vi "RemoveNode.vi"(8 "error in (no error)":errorcluster, 9 "position":T1, 11 "LinkedList in":refnum<class "LinkedList.lvclass">) -> (0 "error out":errorcluster, 1 "ignored":bool, 2 "RemovedNode":refnum<data-value>, 3 "LinkedList out":refnum<class "LinkedList.lvclass">)   [LabVIEW 2013, in "LinkedList.lvclass"]
doc: "Removes a single node from a linked list. If you choose the search option, you must override the IsGoalNode.vi to choose which node to remove."
uses:
  LinkedList.lvclass
  position.ctl
  LLNode/LLNode.lvclass
  LinkedList.lvclass/LinkedList.ctl
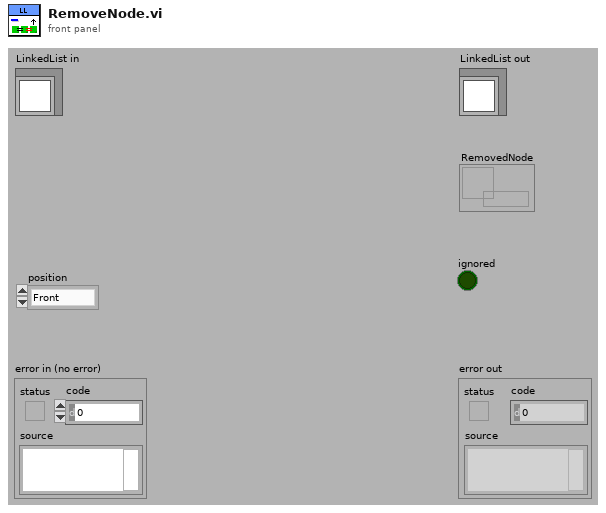
[diagram p1: front panel]
types:
  T1 = typedef "LinkedList.lvclass/position.ctl" = enum16{"Front", "Back", "Search"}
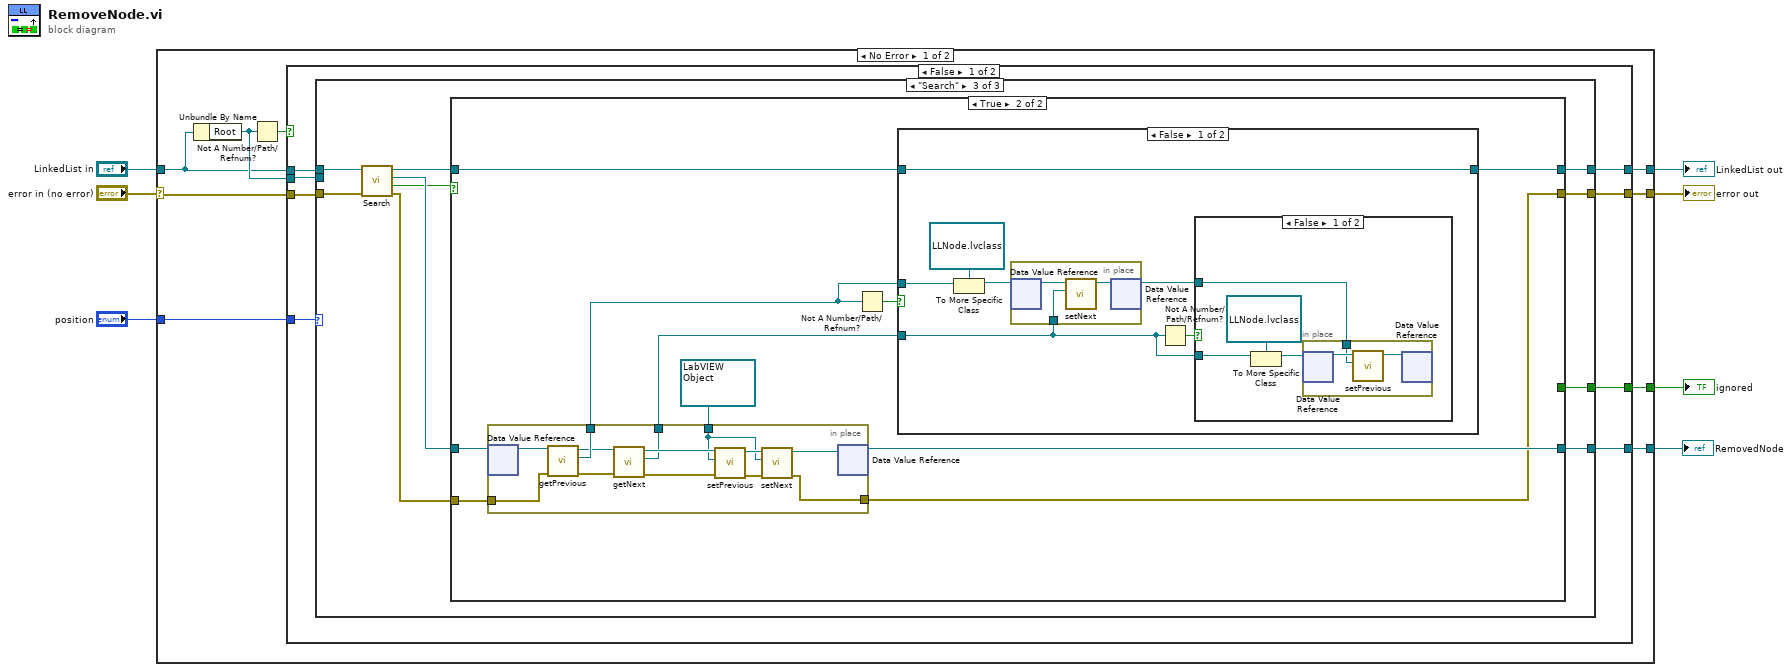
[diagram p0: block diagram]
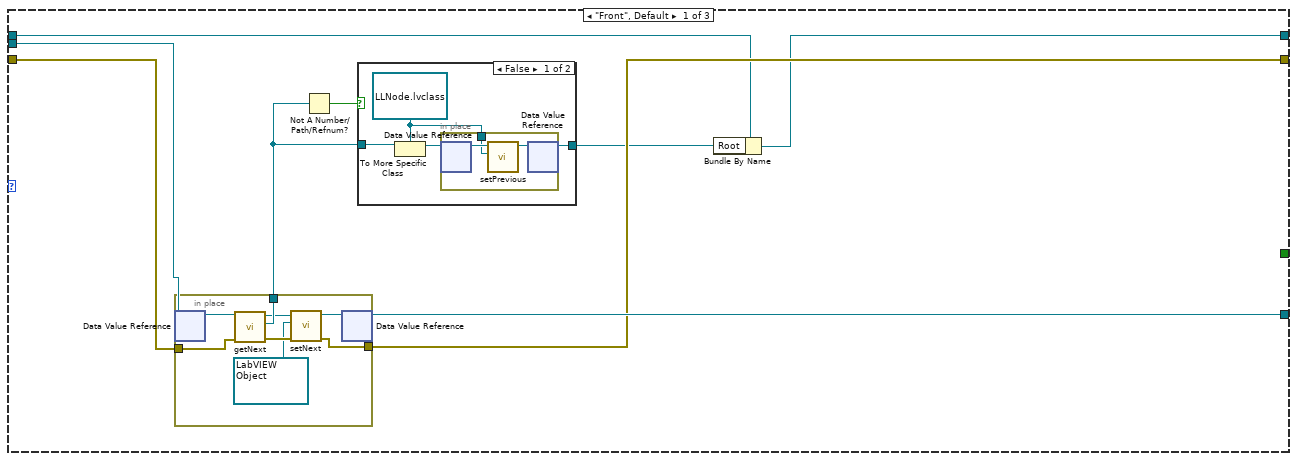
[diagram p2: hidden frame]
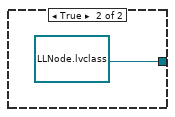
[diagram p3: hidden frame]
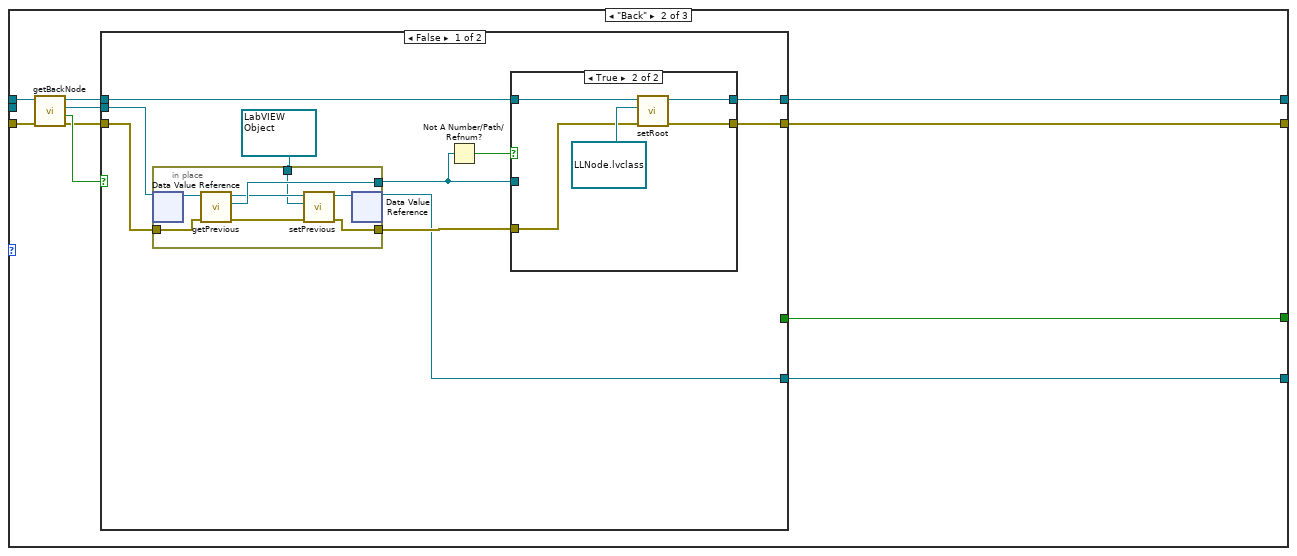
[diagram p4: hidden frame]
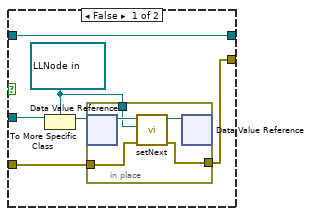
[diagram p5: hidden frame]
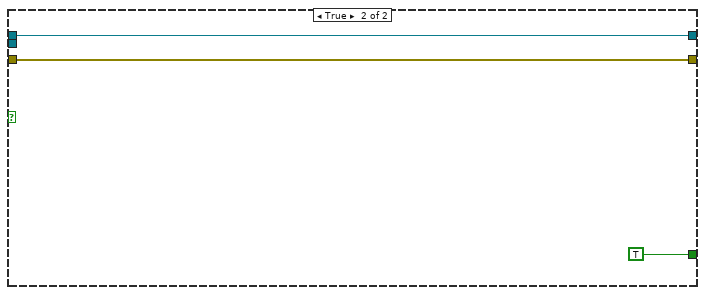
[diagram p6: hidden frame]
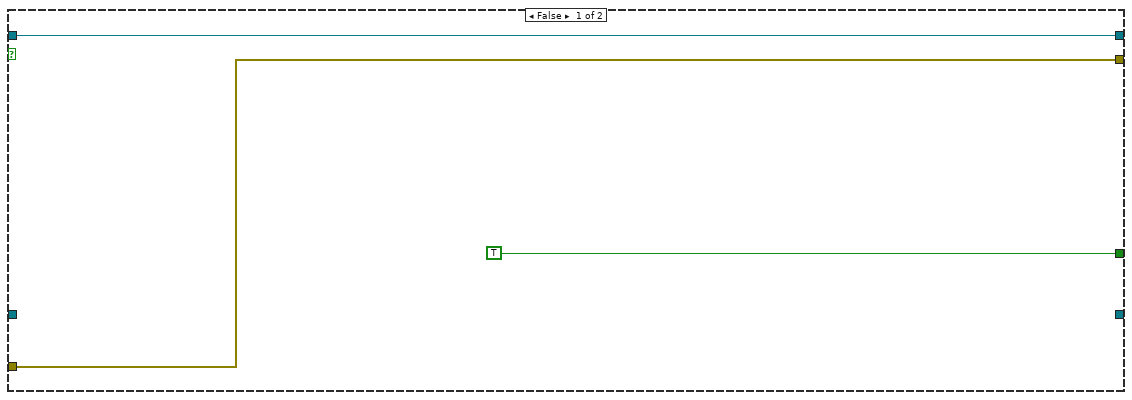
[diagram p7: hidden frame]
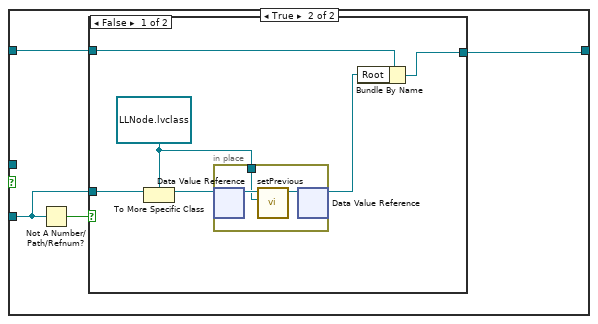
[diagram p9: hidden frame]
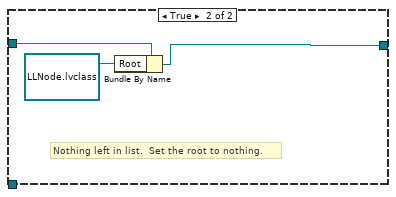
[diagram p10: hidden frame]
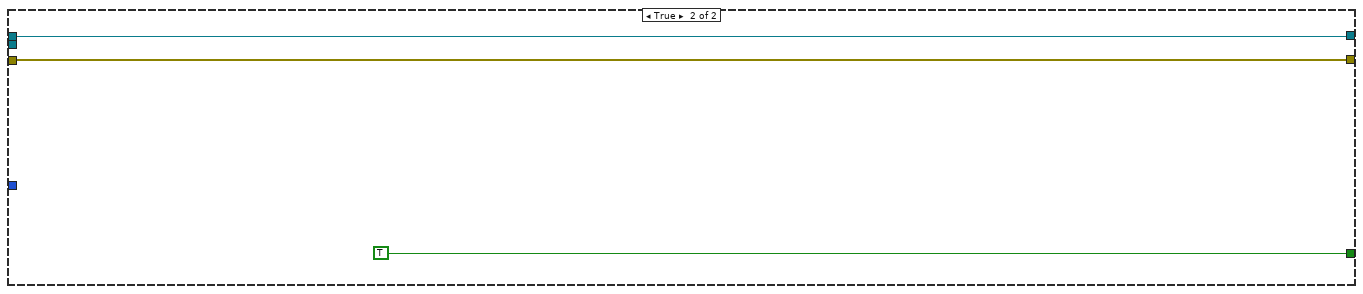
[diagram p11: hidden frame]
diagram:
  n1 = case shown="No Error" "error in (no error)" {
    selector: "error in (no error)" -> [w8 w170]
    tunnel: [w14 w170] -> w6
    tunnel: [w15 w169] -> w4
    tunnel: "LinkedList in" -> [w9 w169]
    tunnel: "position" -> [w16 _]
    tunnel: [w13 _] -> w2
    tunnel: [w12 _] -> w1
    frame No Error {
      n2 = Unbundle By Name(w9) -> ("Root"=w10:refnum<data-value>)
      n3 = Not A Number/Path/Refnum?(number/path/refnum=w10) -> (NaN/Path/Refnum?=w11:bool)
      n4 = case shown="False" w11 {
        tunnel: w16 -> [w24 _]
        tunnel: [w23 TRUE] -> w13
        tunnel: [w22 w168] -> w15
        tunnel: [w21 w167] -> w14
        tunnel: [w20 _] -> w12
        tunnel: w8 -> [w19 w167]
        tunnel: w9 -> [w18 w168]
        tunnel: w10 -> [w17 _]
        frame False {
          n5 = case shown="\"Search\"" w24 {
            tunnel: w18 -> [w27 w59 w102]
            tunnel: [_ w50 w106] -> w23
            tunnel: w19 -> [w32 w56 w100]
            tunnel: [w26 w53 w105] -> w22
            tunnel: [w28 w52 w104] -> w21
            tunnel: [w33 w51 w103] -> w20
            tunnel: w17 -> [w31 _ _]
            frame "Front", Default {
              n6 = in-place {
                in-place-border: w32 -> [w48]
                in-place-border: [w43] -> w28
                in-place-border: [w47] -> w29
                n7 = in-place-dvr #1(w31) -> (w49:refnum<class "LLNode.lvclass">)  [unwired: 1 out]
                n8 = call "getNext.vi"("error in (no error)"=w48, "LLNode in"=w49) -> ("error out"=w44:errorcluster, "next"=w47:refnum<data-value>, "LLNode out"=w46:refnum<class "LLNode.lvclass">)  [unwired: 7 in]
                n9 = call "setNext.vi"("error in (no error)"=w44, "next"=refnum<data-value> refnum ("data value reference"), "LLNode in"=w46) -> ("error out"=w43:errorcluster, "LLNode out"=w45:refnum<class "LLNode.lvclass">)  [unwired: 7 in]
                n10 = in-place-dvr #1(w45) -> (w33:refnum<data-value>)  [unwired: 1 out]
              }
              n11 = Not A Number/Path/Refnum?(number/path/refnum=w29) -> (NaN/Path/Refnum?=w30:bool)
              n12 = case shown="False" w30 {
                tunnel: w29 -> [w37 _]
                tunnel: [w35 refnum<data-value> refnum ("Root")] -> w25
                frame False {
                  w34 = refnum<data-value> refnum ("y")
                  n13 = To More Specific Class(target class=w34, reference=w37) -> (specific class reference=w36:refnum<data-value>)  [unwired: 1 in, 1 out]
                  n14 = in-place {
                    in-place-border: w34 -> [w38]
                    n15 = in-place-dvr #2(w36) -> (w40:refnum<class "LLNode.lvclass">)  [unwired: 1 out]
                    n16 = call "setPrevious.vi"("previous"=w38, "LLNode in"=w40) -> ("LLNode out"=w39:refnum<class "LLNode.lvclass">)  [unwired: 8 in, 1 out]
                    n17 = in-place-dvr #2(w39) -> (w35:refnum<data-value>)  [unwired: 1 out]
                  }
                }
                frame True {
                }
              }
              n18 = Bundle By Name(cluster=w27, "Root"=w25) -> (w26:refnum<class "LinkedList.lvclass">)
            }
            frame "Back" {
              n19 = call "getBackNode.vi"("error in (no error)"=w56, "LinkedList in"=w59) -> ("error out"=w54:errorcluster, "ignore"=w58:bool, "BackNode"=w55:refnum<data-value>, "LinkedList out"=w57:refnum<class "LinkedList.lvclass">)  [unwired: 6 in]
              n20 = case shown="False" w58 {
                tunnel: w57 -> [w67 w95]
                tunnel: w55 -> [w69 _]
                tunnel: w54 -> [w68 w94]
                tunnel: [w65 w95] -> w53
                tunnel: [w64 w94] -> w52
                tunnel: [w63 _] -> w51
                tunnel: [_ TRUE] -> w50
                frame False {
                  n21 = in-place {
                    in-place-border: w68 -> [w87]
                    in-place-border: [w89] -> w66
                    in-place-border: [w93] -> w62
                    in-place-border: refnum<data-value> refnum ("data value reference") -> [w86]
                    n22 = in-place-dvr #3(w69) -> (w92:refnum<class "LLNode.lvclass">)  [unwired: 1 out]
                    n23 = call "getPrevious.vi"("error in (no error)"=w87, "LLNode in"=w92) -> ("error out"=w88:errorcluster, "previous"=w93:refnum<data-value>, "LLNode out"=w91:refnum<class "LLNode.lvclass">)  [unwired: 7 in]
                    n24 = call "setPrevious.vi"("error in (no error)"=w88, "previous"=w86, "LLNode in"=w91) -> ("error out"=w89:errorcluster, "LLNode out"=w90:refnum<class "LLNode.lvclass">)  [unwired: 7 in]
                    n25 = in-place-dvr #3(w90) -> (w63:refnum<data-value>)  [unwired: 1 out]
                  }
                  n26 = Not A Number/Path/Refnum?(number/path/refnum=w62) -> (NaN/Path/Refnum?=w61:bool)
                  n27 = case shown="True" w61 {
                    tunnel: w67 -> [w74 w85]
                    tunnel: w62 -> [w75 _]
                    tunnel: w66 -> [w71 w82]
                    tunnel: [w74 w83] -> w65
                    tunnel: [w70 w81] -> w64
                    frame False {
                      w72 = refnum<data-value> refnum ("BackNode")
                      n28 = To More Specific Class(target class=w72, reference=w75) -> (specific class reference=w73:refnum<data-value>)  [unwired: 1 in, 1 out]
                      n29 = in-place {
                        in-place-border: w72 -> [w78]
                        in-place-border: w71 -> [w77]
                        in-place-border: [w76] -> w70
                        n30 = in-place-dvr #4(w73) -> (w80:refnum<class "LLNode.lvclass">)  [unwired: 1 out]
                        n31 = call "setNext.vi"("error in (no error)"=w77, "next"=w78, "LLNode in"=w80) -> ("error out"=w76:errorcluster, "LLNode out"=w79:refnum<class "LLNode.lvclass">)  [unwired: 7 in]
                        n32 = in-place-dvr #4(w79) -> ()  [unwired: 2 out]
                      }
                    }
                    frame True {
                      n33 = call "setRoot.vi"("error in (no error)"=w82, "Root"=refnum<data-value> refnum, "LinkedList in"=w85) -> ("error out"=w81:errorcluster, "LinkedList out"=w83:refnum<class "LinkedList.lvclass">)  [unwired: 7 in]
                    }
                  }
                }
                frame True {
                }
              }
            }
            frame "Search" {
              n34 = call "Search.vi"("error in (no error)"=w100, "LinkedList in"=w102) -> ("error out"=w99:errorcluster, "found"=w97:bool, "Node"=w98:refnum<data-value>, "LinkedList out"=w101:refnum<class "LinkedList.lvclass">)  [unwired: 6 in]
              n35 = case shown="True" w97 {
                tunnel: w101 -> [w108 w119]
                tunnel: w98 -> [_ w117]
                tunnel: w99 -> [w107 w112]
                tunnel: [TRUE _] -> w106
                tunnel: [w108 w118] -> w105
                tunnel: [w107 w110] -> w104
                tunnel: [_ w111] -> w103
                frame False {
                }
                frame True {
                  n36 = in-place {
                    in-place-border: [w164] -> w113
                    in-place-border: refnum<data-value> refnum ("data value reference") -> [w159]
                    in-place-border: [w158] -> w114
                    in-place-border: w112 -> [w157]
                    in-place-border: [w153] -> w110
                    n37 = in-place-dvr #5(w117) -> (w165:refnum<class "LLNode.lvclass">)  [unwired: 1 out]
                    n38 = call "getPrevious.vi"("error in (no error)"=w157, "LLNode in"=w165) -> ("error out"=w156:errorcluster, "previous"=w164:refnum<data-value>, "LLNode out"=w163:refnum<class "LLNode.lvclass">)  [unwired: 7 in]
                    n39 = call "getNext.vi"("error in (no error)"=w156, "LLNode in"=w163) -> ("error out"=w155:errorcluster, "next"=w158:refnum<data-value>, "LLNode out"=w161:refnum<class "LLNode.lvclass">)  [unwired: 7 in]
                    n40 = call "setPrevious.vi"("error in (no error)"=w155, "previous"=w159, "LLNode in"=w161) -> ("error out"=w154:errorcluster, "LLNode out"=w160:refnum<class "LLNode.lvclass">)  [unwired: 7 in]
                    n41 = call "setNext.vi"("error in (no error)"=w154, "next"=w159, "LLNode in"=w160) -> ("error out"=w153:errorcluster, "LLNode out"=w162:refnum<class "LLNode.lvclass">)  [unwired: 7 in]
                    n42 = in-place-dvr #5(w162) -> (w111:refnum<data-value>)  [unwired: 1 out]
                  }
                  n43 = Not A Number/Path/Refnum?(number/path/refnum=w113) -> (NaN/Path/Refnum?=w115:bool)
                  n44 = case shown="False" w115 {
                    tunnel: w119 -> [w121 w138]
                    tunnel: [w121 w137] -> w118
                    tunnel: w114 -> [w122 w139]
                    tunnel: w113 -> [w126 _]
                    frame False {
                      n45 = To More Specific Class(target class=refnum<data-value> refnum ("LLNode out"), reference=w126) -> (specific class reference=w124:refnum<data-value>)  [unwired: 1 in, 1 out]
                      n46 = in-place {
                        in-place-border: w122 -> [w134]
                        n47 = in-place-dvr #6(w124) -> (w135:refnum<class "LLNode.lvclass">)  [unwired: 1 out]
                        n48 = call "setNext.vi"("next"=w134, "LLNode in"=w135) -> ("LLNode out"=w136:refnum<class "LLNode.lvclass">)  [unwired: 8 in, 1 out]
                        n49 = in-place-dvr #6(w136) -> (w120:refnum<data-value>)  [unwired: 1 out]
                      }
                      n50 = Not A Number/Path/Refnum?(number/path/refnum=w122) -> (NaN/Path/Refnum?=w123:bool)
                      n51 = case shown="False" w123 {
                        tunnel: w122 -> [w129 _]
                        tunnel: w120 -> [w127 _]
                        frame False {
                          n52 = To More Specific Class(target class=refnum<data-value> refnum ("LLNode out"), reference=w129) -> (specific class reference=w128:refnum<data-value>)  [unwired: 1 in, 1 out]
                          n53 = in-place {
                            in-place-border: w127 -> [w131]
                            n54 = in-place-dvr #7(w128) -> (w133:refnum<class "LLNode.lvclass">)  [unwired: 1 out]
                            n55 = call "setPrevious.vi"("previous"=w131, "LLNode in"=w133) -> ("LLNode out"=w132:refnum<class "LLNode.lvclass">)  [unwired: 8 in, 1 out]
                            n56 = in-place-dvr #7(w132) -> ()  [unwired: 2 out]
                          }
                        }
                        frame True {
                        }
                      }
                    }
                    frame True {
                      n57 = Not A Number/Path/Refnum?(number/path/refnum=w139) -> (NaN/Path/Refnum?=w140:bool)
                      n58 = case shown="False" w140 {
                        tunnel: w139 -> [w146 _]
                        tunnel: w138 -> [w143 w152]
                        tunnel: [w141 w150] -> w137
                        frame False {
                          w144 = refnum<data-value> refnum ("LLNode out")
                          n59 = To More Specific Class(target class=w144, reference=w146) -> (specific class reference=w145:refnum<data-value>)  [unwired: 1 in, 1 out]
                          n60 = in-place {
                            in-place-border: w144 -> [w147]
                            n61 = in-place-dvr #8(w145) -> (w149:refnum<class "LLNode.lvclass">)  [unwired: 1 out]
                            n62 = call "setPrevious.vi"("previous"=w147, "LLNode in"=w149) -> ("LLNode out"=w148:refnum<class "LLNode.lvclass">)  [unwired: 8 in, 1 out]
                            n63 = in-place-dvr #8(w148) -> (w142:refnum<data-value>)  [unwired: 1 out]
                          }
                          n64 = Bundle By Name(cluster=w143, "Root"=w142) -> (w141:refnum<class "LinkedList.lvclass">)
                        }
                        frame True {
                          # "Nothing left in list.  Set the root to nothing."
                          n65 = Bundle By Name(cluster=w152, "Root"=refnum<data-value> refnum) -> (w150:refnum<class "LinkedList.lvclass">)
                        }
                      }
                    }
                  }
                }
              }
            }
          }
        }
        frame True {
        }
      }
    }
    frame Error {
    }
  }
  "error out" <- w6
  "LinkedList out" <- w4
  "RemovedNode" <- w1
  "ignored" <- w2
